vi "Read Temperatures DBL.vi"(8 "error in":errorcluster, 10 "Source":string, 11 "IRead Temperatures Multichannel in":refnum<class "DAQmx Thermocouple Continuous Read Strategy.lvclass">) -> (0 "error out":errorcluster, 1 "Timestamps":timestamp[](array[timestamp]) format="%<%x %.3X>T", 2 "Temperatures":dbl[](array[numeric]), 3 "IRead Temperatures Multichannel out":refnum<class "DAQmx Thermocouple Continuous Read Strategy.lvclass">)   [LabVIEW 2024, in "DAQmx Thermocouple Continuous Read Strategy.lvclass"]
uses:
  DAQmx Thermocouple Continuous Read Strategy.lvclass
  DAQmx Base Configure Strategy/DAQmx Base Configure Strategy.lvclass
  <vilib>/DAQmx/read.llb/DAQmx Read (Analog 2D DBL NChan NSamp).vi
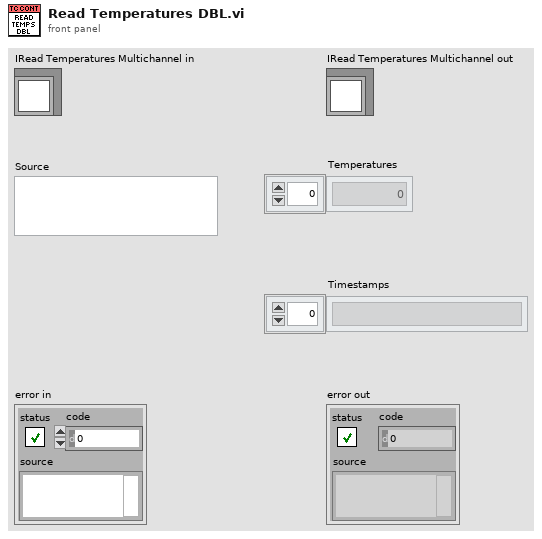
[diagram p1: front panel]
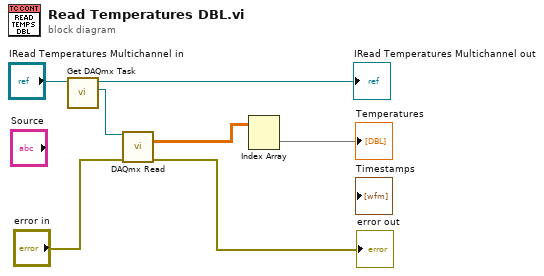
[diagram p0: block diagram]
diagram:
  n1 = call "Get DAQmx Task.vi"("DAQmx Base Configure Strategy in"="IRead Temperatures Multichannel in") -> ("DAQmx Task"=w3:refnum<k21>, "DAQmx Base Configure Strategy out"=→"IRead Temperatures Multichannel out":refnum<class "DAQmx Thermocouple Continuous Read Strategy.lvclass">)  [unwired: 9 in]
  n2 = call-poly <vilib>:"DAQmx Read.vi"("task/channels in"=w3, "error in"="error in") -> ("data"=w2:dbl[][], "error out"=→"error out":errorcluster)  [unwired: 11 in, 1 out]
  n3 = Index Array(array=w2) -> (element=→"Temperatures":dbl[])  [unwired: 2 in]
